vi "Channel 2 DAQMx Channel.vi"(10 "Channel In":string) -> (1 "DAQmx Task":refnum<k21>, 2 "DAQmx Channel":refnum<k21>)   [LabVIEW 2013]
uses:
  Data Access Objects/Metadata/Persistant DAO Actions.ctl
  <resource>/objmgr/daqmx.rc
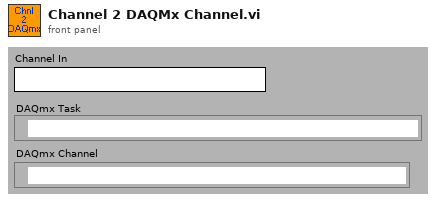
[diagram p1: front panel]
types:
  T1 = typedef "Persistant DAO Actions.ctl" = enum16{"Init", "Get", "Set", "Load", "Save"}
  T2 = typedef "DAQMx Tasks.ctl" = cluster{"LBCB1 Readings":refnum<k21>, "LBCB2 Readings":refnum<k21>, "LBCB1 Commands":refnum<k21>, "LBCB2 Commands":refnum<k21>, "Sensors":refnum<k21>[]}
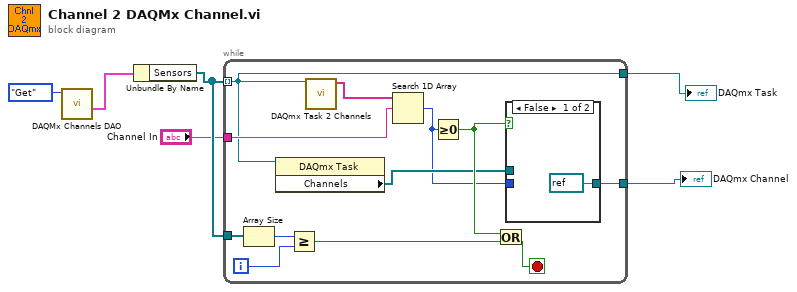
[diagram p0: block diagram]
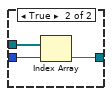
[diagram p2: hidden frame]
diagram:
  n1 = call "DAQMx Channels DAO.vi"("Actions"=Persistant_DAO_Actions."Get") -> ("Names Out"=w5:T2)  [unwired: 8 in, 2 out]
  n2 = Unbundle By Name(w5) -> ("Sensors"=w4:refnum<k21>[])
  n3 = while {
    tunnel: w4 -> [w11] mode=indexing
    tunnel: w4 -> [w18]
    tunnel: "Channel In" -> [w13]
    tunnel: [w11] -> w2
    tunnel: [w7] -> w1
    i -> [w16]
    stop <- w12 stop-if-true
    n4 = Array Size(array=w18) -> (size(s)=w17:i32)
    n5 = property class="DAQmx Task"(reference=w11) -> ("Channels"=w9:refnum<k21>[])  [unwired: 1 in, 2 out]
    n6 = Greater Or Equal?(x=w17, y=w16) -> (x >= y?=w15:bool)
    n7 = call "DAQmx Task 2 Channels.vi"("DAQmx Task Name"=w11) -> ("Channels Out"=w14:string[])  [unwired: 10 in]
    n8 = Search 1D Array(1D array=w14, element=w13) -> (index of element=w8:i32)  [unwired: 1 in]
    n9 = Greater Or Equal To 0?(x=w8) -> (x >= 0?=w10:bool)
    n10 = Or(x=w10, y=w15) -> (x .or. y?=w12:bool)
    n11 = case shown="False" w10 {
      tunnel: w9 -> [_ w22]
      tunnel: w8 -> [_ w21]
      tunnel: [refnum<k21> refnum w20] -> w7
      frame False {
      }
      frame True {
        n12 = Index Array(array=w22, index=w21) -> (element=w20:refnum<k21>)
      }
    }
  }
  "DAQmx Task" <- w2
  "DAQmx Channel" <- w1
